vi "get IR test parameters.vi"(8 "error in (no error)":errorcluster, 10 "Step":T2 min=1 max=99 step=1, 11 "VISA Refnum in":refnum<visa-resource-name>) -> (0 "error out":errorcluster, 3 "VISA Refnum out":refnum<visa-resource-name>, 5 "IR Parameters":T1 {"Voltage Level [V]" format="%.3p"; "Hi Limit [ohm]" format="%#_6p"; "Lo Limit [ohm]" format="%#_6p"})   [LabVIEW 2025]
uses:
  Type Def/steps--ring.ctl
  Type Def/AC-DC-IR modes--ring.ctl
  Type Def/DC-IR modes--ring.ctl
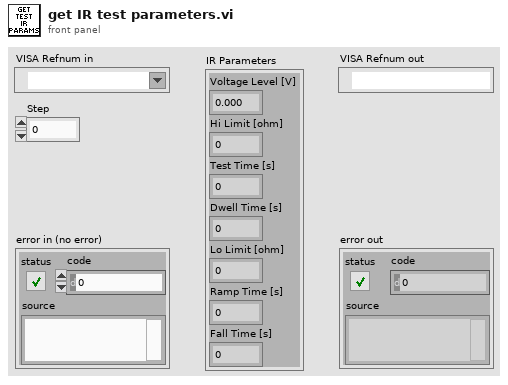
[diagram p1: front panel]
types:
  T1 = cluster{"Voltage Level [V]":u16, "Hi Limit [ohm]":dbl, "Test Time [s] ":dbl, "Dwell Time [s]":dbl, "Lo Limit [ohm]":dbl, "Ramp Time [s] ":dbl, "Fall Time [s]":dbl}
  T2 = typedef "steps--ring.ctl" = u8
  T3 = typedef "DC-IR modes--ring.ctl" = u16
  T4 = typedef "AC-DC-IR modes--ring.ctl" = u16
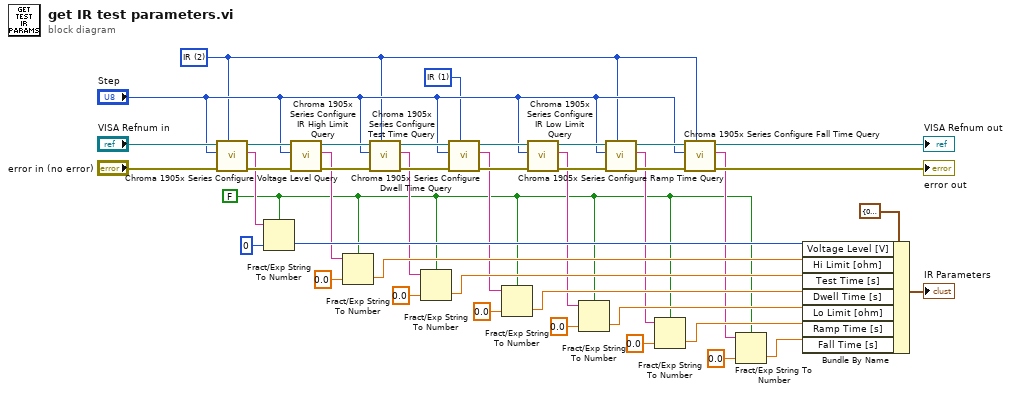
[diagram p0: block diagram]
diagram:
  w1 = FALSE ("use system decimal point (T)")
  w26 = T3 1 items=["DC", "IR"] ("Mode")
  w25 = T4 2 items=["AC", "DC", "IR"] ("Mode")
  n1 = call "Chroma 1905x Series Configure Voltage Level Query.vi"("Mode"=w25, "error in (no error)"="error in (no error)", "Step"="Step", "VISA resource name"="VISA Refnum in") -> ("error out"=w34:errorcluster, "Voltage value [V]"=w22:string, "VISA resource name out"=w31:refnum<visa-resource-name>)  [unwired: 5 in]
  n2 = Fract/Exp String To Number(use system decimal point (T)=w1, string=w22, default (0 dbl)=u16 0 ("Voltage Level [V]")) -> (number=w20:u16)  [unwired: 1 in, 1 out]
  n3 = call "Chroma 1905x Series Configure IR High Limit Query.vi"("error in (no error)"=w34, "Step"="Step", "VISA resource name"=w31) -> ("error out"=w37:errorcluster, "IR Hi limit value [ohm]"=w18:string, "VISA resource name out"=w38:refnum<visa-resource-name>)  [unwired: 6 in]
  n4 = Fract/Exp String To Number(use system decimal point (T)=w1, string=w18, default (0 dbl)=0.0 ("Voltage Level [V]")) -> (number=w17:dbl)  [unwired: 1 in, 1 out]
  n5 = call "Chroma 1905x Series Configure Test Time Query.vi"("Mode"=w25, "error in (no error)"=w37, "Step"="Step", "VISA resource name"=w38) -> ("error out"=w40:errorcluster, "Test Time value [s]"=w15:string, "VISA resource name out"=w28:refnum<visa-resource-name>)  [unwired: 5 in]
  n6 = Fract/Exp String To Number(use system decimal point (T)=w1, string=w15, default (0 dbl)=0.0 ("Voltage Level [V]")) -> (number=w14:dbl)  [unwired: 1 in, 1 out]
  n7 = call "Chroma 1905x Series Configure Dwell Time Query.vi"("Mode"=w26, "error in (no error)"=w40, "Step"="Step", "VISA resource name"=w28) -> ("error out"=w39:errorcluster, "Dwell time value [s]"=w12:string, "VISA resource name out"=w41:refnum<visa-resource-name>)  [unwired: 5 in]
  n8 = Fract/Exp String To Number(use system decimal point (T)=w1, string=w12, default (0 dbl)=0.0 ("Voltage Level [V]")) -> (number=w11:dbl)  [unwired: 1 in, 1 out]
  n9 = call "Chroma 1905x Series Configure IR Low Limit Query.vi"("error in (no error)"=w39, "Step"="Step", "VISA resource name"=w41) -> ("error out"=w43:errorcluster, "IR Lo limit value [ohm]"=w9:string, "VISA resource name out"=w42:refnum<visa-resource-name>)  [unwired: 6 in]
  n10 = Fract/Exp String To Number(use system decimal point (T)=w1, string=w9, default (0 dbl)=0.0 ("Voltage Level [V]")) -> (number=w8:dbl)  [unwired: 1 in, 1 out]
  n11 = call "Chroma 1905x Series Configure Ramp Time Query.vi"("Mode"=w25, "error in (no error)"=w43, "Step"="Step", "VISA resource name"=w42) -> ("error out"=w35:errorcluster, "Ramp Time value [s]"=w6:string, "VISA resource name out"=w36:refnum<visa-resource-name>)  [unwired: 5 in]
  n12 = Fract/Exp String To Number(use system decimal point (T)=w1, string=w6, default (0 dbl)=0.0 ("Voltage Level [V]")) -> (number=w5:dbl)  [unwired: 1 in, 1 out]
  n13 = call "Chroma 1905x Series Configure Fall Time Query.vi"("Mode"=w25, "error in (no error)"=w35, "Step"="Step", "VISA resource name"=w36) -> ("error out"=→"error out":errorcluster, "Fall Time value"=w3:string, "VISA resource name out"=→"VISA Refnum out":refnum<visa-resource-name>)  [unwired: 5 in]
  n14 = Fract/Exp String To Number(use system decimal point (T)=w1, string=w3, default (0 dbl)=0.0 ("Voltage Level [V]")) -> (number=w2:dbl)  [unwired: 1 in, 1 out]
  n15 = Bundle By Name(cluster=T1 {"Voltage Level [V]"=0, "Hi Limit [ohm]"=0.0, "Test Time [s] "=0.0, "Dwell Time [s]"=0.0, "Lo Limit [ohm]"=0.0, "Ramp Time [s] "=0.0, "Fall Time [s]"=0.0} ("IR Parameters"), "Voltage Level [V]"=w20, "Hi Limit [ohm]"=w17, "Test Time [s]"=w14, "Dwell Time [s]"=w11, "Lo Limit [ohm]"=w8, "Ramp Time [s]"=w5, "Fall Time [s]"=w2) -> (→"IR Parameters":T1)
